vi "主画面_古田污水厂.vi"() -> ()   [LabVIEW 2016]
uses:
  <vilib>/Utility/config.llb/Read Key (String).vi
  <vilib>/Utility/config.llb/NI_LVConfig.lvlib
  PLC/PLC.lvlib
  data/FreeMem.dll
panel:
  in  "全屏":T1
  out "站点名称":string="站点名称"
  out "时间显示":string="2017-05-09 10:50:42"
  out "Version":string="Version:1.0.0"
  in  "主画面菜单":enum32{"首页", "数据查询", "运维调试", "系统设置"}(xcontrol)
  # "一体化微 型 水 质 监 测 站"
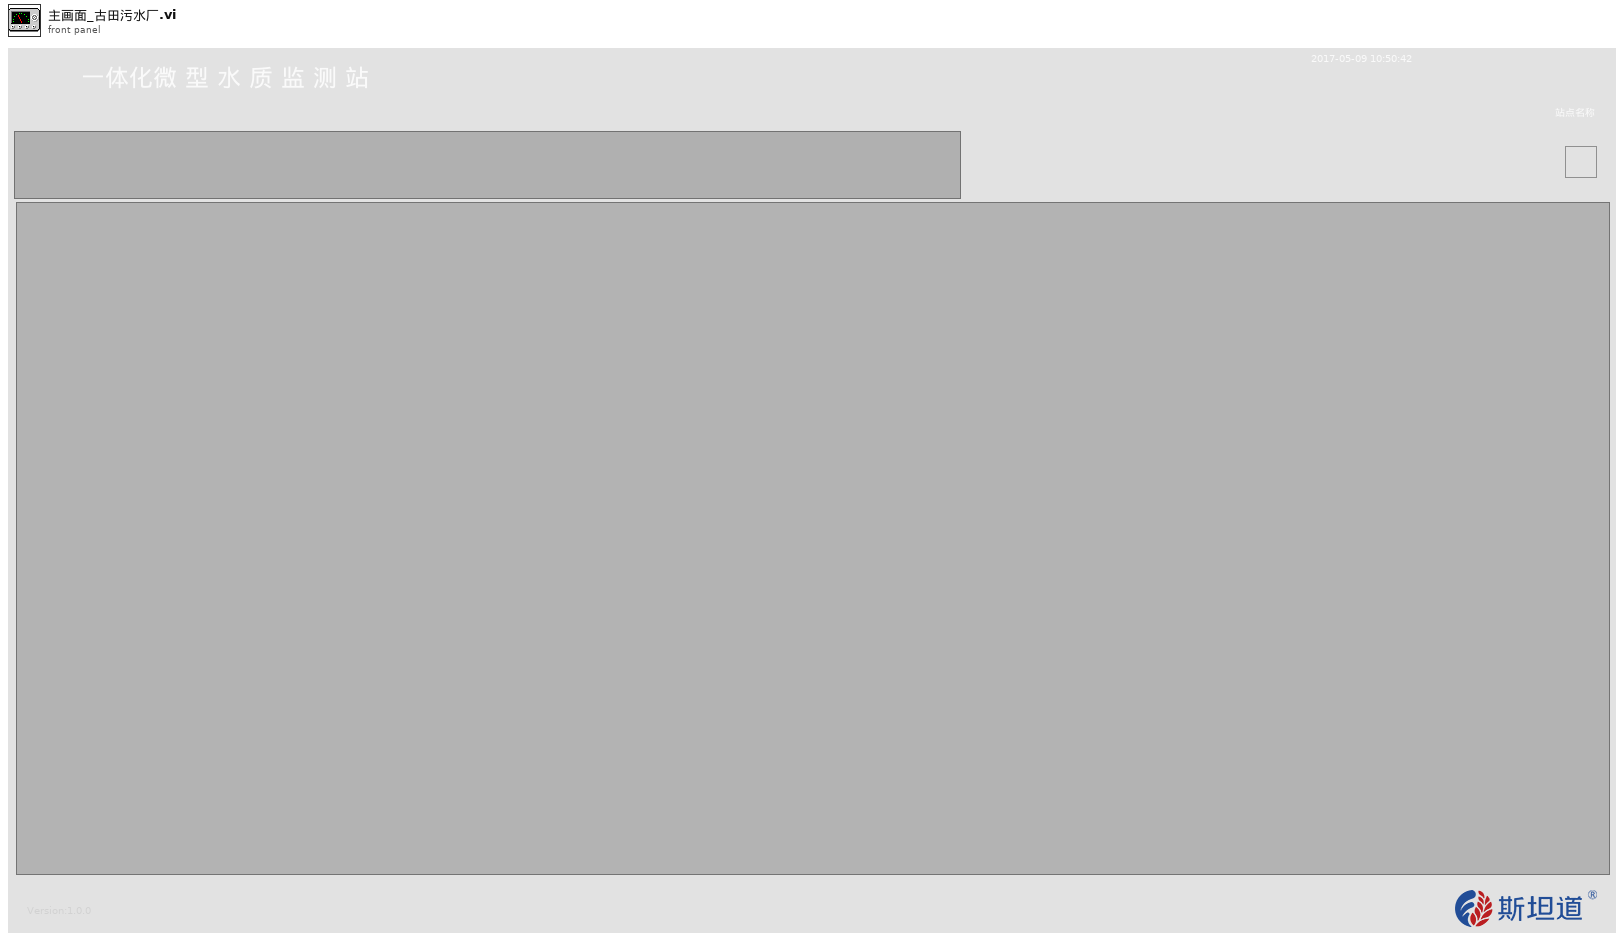
[diagram p1: front panel]
types:
  T1 = typedef "全屏按钮.ctl" = bool
  T2 = cluster{"时间标识":timestamp, "设备":string, "日志信息":string, "流程参数":string}
  T3 = enum32{"invalid app kind", "Development System", "Run Time System", "Student Edition", "Embedded LabVIEW", "Evaluation", "Custom"}
  T4 = typedef "NI_LVConfig.lvlib/Config Data RefNum.ctl" = refnum<k1>
  T5 = cluster{"Y0":bool, "Y1":bool, "Y2":bool, "Y3":bool, "Y4":bool, "Y5":bool, "Y6":bool, "Y7":bool, "Y8":bool, "Y9":bool, "Y10":bool, "Y11":bool, "Y12":bool, "Y13":bool, "Y14":bool, "Y15":bool}
  T6 = enum32{"Bad", "Idle", "Run top level", "Running"}
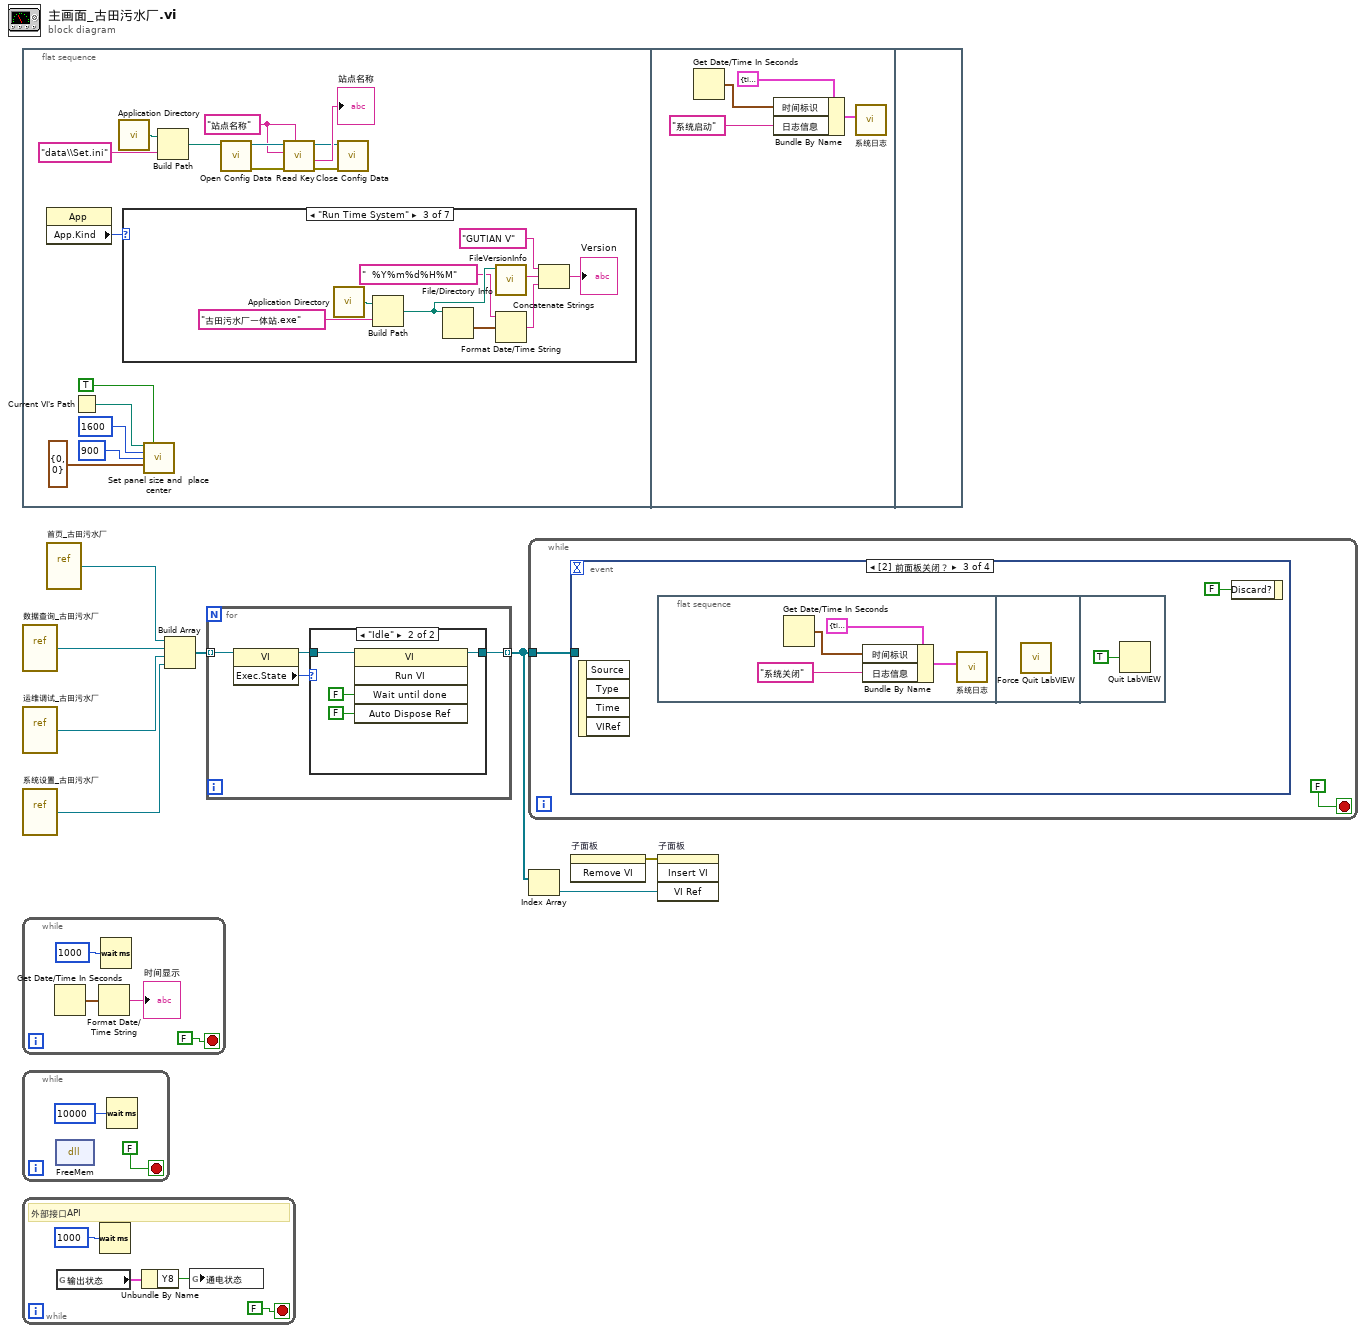
[diagram p0: block diagram]
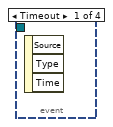
[diagram p9: hidden frame]
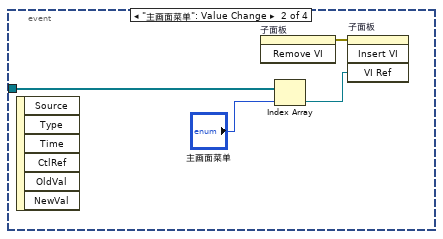
[diagram p10: hidden frame]
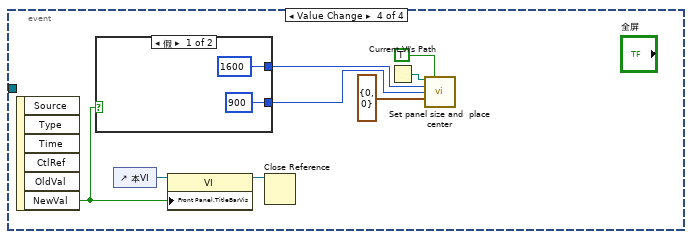
[diagram p11: hidden frame]
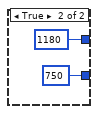
[diagram p12: hidden frame]
diagram:
  n1 = flat-sequence {
    frame #0 {
      w9 = "站点名称" ("section")
      n2 = property class="App"() -> ("App.Kind"=w20:T3)  [unwired: 2 in, 2 out]
      n3 = Current VI's Path() -> (path=w23:path)
      n4 = call <vilib>:"Application Directory.vi"() -> ("Application Directory"=w12:path)
      n5 = case shown="\"Run Time System\"" w20 {
        frame "invalid app kind" {
        }
        frame "Development System", Default {
        }
        frame "Run Time System" {
          n6 = call <vilib>:"Application Directory.vi"() -> ("Application Directory"=w31:path)
          n7 = Build Path(base path=w31, name or relative path="古田污水厂一体站.exe" ("名称或相对路径")) -> (appended path=w27:path)
          n8 = File/Directory Info(path=w27) -> (last mod=w26:timestamp)  [unwired: 1 in, 6 out]
          n9 = call <vilib>:"FileVersionInfo.vi"("Application Path in"=w27) -> ("File Version Info"=w29:string)  [unwired: 7 in, 3 out]
          n10 = Format Date/Time String(time format string (%c)="  %Y%m%d%H%M" ("时间格式字符串(%c)"), seconds (now)=w26) -> (date/time string=w24:string)  [unwired: 1 in]
          n11 = Concatenate Strings("GUTIAN V" ("字符串"), w29, w24) -> (→"Version":string)
        }
        frame "Student Edition" {
        }
        frame "Embedded LabVIEW" {
        }
        frame "Evaluation" {
        }
        frame "Custom" {
        }
      }
      n12 = call "Set panel size and  place center.vi"("Path"=w23, "Close Reference (false)"=TRUE, "Panel Width"=1600, "Panel Height"=900, "FP.Origin in(H & V)"=cluster{"Horizontal":i16, "Vertical":i16} {"Horizontal"=0, "Vertical"=0}) -> ()  [unwired: 6 in, 5 out]
      n13 = Build Path(base path=w12, name or relative path="data\\Set.ini" ("名称或相对路径")) -> (appended path=w10:path)
      n14 = call <vilib>:"Open Config Data.vi"("configuration file path"=w10) -> ("error out"=w14:errorcluster, "refnum"=w17:T4)  [unwired: 8 in, 1 out]
      n15 = call-poly <vilib>:"Read Key.vi"("section"=w9, "error in (no error)"=w14, "key"=w9, "refnum"=w17) -> ("error out"=w13:errorcluster, "value"=→"站点名称":string, "refnum out"=w15:T4)  [unwired: 4 in, 1 out]
      n16 = call <vilib>:"Close Config Data.vi"("error in (no error)"=w13, "refnum"=w15) -> ()  [unwired: 8 in, 2 out]
    }
    frame #1 {
      n17 = Get Date/Time In Seconds() -> (seconds since 1Jan1904=w34:timestamp)
      n18 = Bundle By Name(cluster=T2 {"时间标识"=timestamp(0 s since 1904-01-01), "设备"="系统", "日志信息"="", "流程参数"=""} ("data in"), "时间标识"=w34, "日志信息"="系统启动") -> (w35:T2)
      n19 = call "系统日志.vi"("data in"=w35) -> ()  [unwired: 11 in]
    }
    frame #2 {
    }
  }
  n20 = vi-ref "数据查询_古田污水厂.vi"() -> (w4:refnum<vi>)
  n21 = vi-ref "运维调试_古田污水厂.vi"() -> (w3:refnum<vi>)
  n22 = vi-ref "系统设置_古田污水厂.vi"() -> (w2:refnum<vi>)
  n23 = while {
    stop <- FALSE stop-if-true
    n24 = Get Date/Time In Seconds() -> (seconds since 1Jan1904=w37:timestamp)
    n25 = Format Date/Time String(seconds (now)=w37) -> (date/time string=→"时间显示":string)  [unwired: 2 in]
    n26 = Wait (ms)(milliseconds to wait=u32 1000 ("等待时间（毫秒）")) -> ()  [unwired: 1 out]
  }
  n27 = while {
    stop <- FALSE stop-if-true
    n28 = dll-call lib="PTH2sabs CUsersHsiao\nSynologyDrive工作资料\t待发货古田项目GT一体站项目dataFreeMem.dll" fn="FreeMem"() -> ()  [unwired: 4 in, 2 out]
    n29 = Wait (ms)(milliseconds to wait=u32 10000 ("等待时间（毫秒）")) -> ()  [unwired: 1 out]
  }
  n30 = while "While循环" {
    stop <- FALSE stop-if-true
    # "外部接口API"
    n31 = global read "采配水全局变量.vi" "输出状态"() -> (w46:T5)
    n32 = Wait (ms)(milliseconds to wait=u32 1000 ("等待时间（毫秒）")) -> ()  [unwired: 1 out]
    n33 = Unbundle By Name(w46) -> ("Y8"=w45:bool)
    n34 = global write "多参数全局变量.vi" "通电状态"(w45) -> ()
  }
  n35 = vi-ref "首页_古田污水厂.vi"() -> (w5:refnum<vi>)
  n36 = Build Array(w5, w4, w3, w2) -> (w1:refnum<vi>[])
  n37 = for {
    tunnel: w1 -> [w50] mode=indexing
    tunnel: [w47] -> w7 mode=indexing
    n38 = property class="VI"(reference=w50) -> (reference out=w48:refnum<vi>, "Exec.State"=w49:T6)  [unwired: 1 in, 1 out]
    n39 = case shown="\"Idle\"" w49 {
      tunnel: w48 -> [w51 w53]
      tunnel: [w51 w52] -> w47
      frame "Bad", Default {
      }
      frame "Idle" {
        n40 = invoke class="VI" method="Run VI"(reference=w53, "Wait until done"=FALSE ("结束前等待"), "Auto Dispose Ref"=FALSE ("自动销毁引用")) -> (reference out=w52:refnum<vi>)  [unwired: 2 in, 4 out]
      }
    }
  }
  n41 = while {
    tunnel: w7 -> [w56]
    stop <- FALSE stop-if-true
    n42 = event shown="[2] 前面板关闭？" {
      selector: _ -> [_ _ _ _]
      dyn-events: _ -> [_ _ _ _]
      timeout: _ -> [_ _ _ _]
      tunnel: w56 -> [_ w60 _ _]
      event Timeout {
        n43 = event-data() -> ()  [unwired: 1 in, 3 out]
      }
      event "主画面菜单": Value Change {
        n44 = event-data() -> ()  [unwired: 1 in, 6 out]
        n45 = invoke on="子面板" class="SubPnl" method="Remove VI"() -> (error out=w58:errorcluster)  [unwired: 3 in, 2 out]
        n46 = Index Array(array=w60, index="主画面菜单") -> (element=w59:refnum<vi>)
        n47 = invoke on="子面板" class="SubPnl" method="Insert VI"(error in=w58, "VI Ref"=w59) -> ()  [unwired: 2 in, 4 out]
      }
      event Panel Close? {
        n48 = event-data() -> ()  [unwired: 1 in, 4 out]
        n49 = flat-sequence {
          frame #0 {
            n50 = Get Date/Time In Seconds() -> (seconds since 1Jan1904=w65:timestamp)
            n51 = Bundle By Name(cluster=T2 {"时间标识"=timestamp(0 s since 1904-01-01), "设备"="系统", "日志信息"="", "流程参数"=""} ("data in"), "时间标识"=w65, "日志信息"="系统关闭") -> (w64:T2)
            n52 = call "系统日志.vi"("data in"=w64) -> ()  [unwired: 11 in]
          }
          frame #1 {
            n53 = call "Force Quit LabVIEW.vi"() -> ()  [unwired: 10 in, 2 out]
          }
          frame #2 {
            n54 = Quit LabVIEW(quit? (T)=TRUE ("退出？(T)")) -> ()
          }
        }
        n55 = event-data("Discard?"=FALSE ("放弃？")) -> ()  [unwired: 1 in, 1 out]
      }
      event Value Change {
        n56 = event-data() -> ("NewVal"=w70:T1)  [unwired: 1 in, 5 out]
        n57 = case shown="假" w70 {
          tunnel: [1600 ("Panel Width") 1180 ("Panel Width")] -> w69
          tunnel: [900 ("Panel Height") 750 ("Panel Height")] -> w68
          frame False {
          }
          frame True {
          }
        }
        n58 = control-ref of="本VI"() -> (w75:refnum<vi>)
        n59 = property class="VI"(reference=w75, "Front Panel.TitleBarVis"=w70) -> (reference out=w71:refnum<vi>)  [unwired: 1 in, 1 out]
        n60 = Close Reference(reference=w71) -> ()  [unwired: 1 in, 1 out]
        n61 = Current VI's Path() -> (path=w74:path)
        n62 = call "Set panel size and  place center.vi"("Path"=w74, "Close Reference (false)"=TRUE, "Panel Width"=w69, "Panel Height"=w68, "FP.Origin in(H & V)"=cluster{"Horizontal":i16, "Vertical":i16} {"Horizontal"=0, "Vertical"=0}) -> ()  [unwired: 6 in, 5 out]
      }
    }
  }
  n63 = Index Array(array=w7) -> (element=w6:refnum<vi>)  [unwired: 1 in]
  n64 = invoke on="子面板" class="SubPnl" method="Remove VI"() -> (error out=w8:errorcluster)  [unwired: 3 in, 2 out]
  n65 = invoke on="子面板" class="SubPnl" method="Insert VI"(error in=w8, "VI Ref"=w6) -> ()  [unwired: 2 in, 4 out]
